vi "Base_Init.vi"(8 "error in (no error)":errorcluster, 10 "String":string, 11 "object in":refnum<class "Base.lvclass">) -> (0 "error out":errorcluster, 3 "object out":refnum<class "Base.lvclass">)   [LabVIEW 2019, in "Base.lvclass"]
uses:
  Base.lvclass
  Base.lvclass/Base.ctl
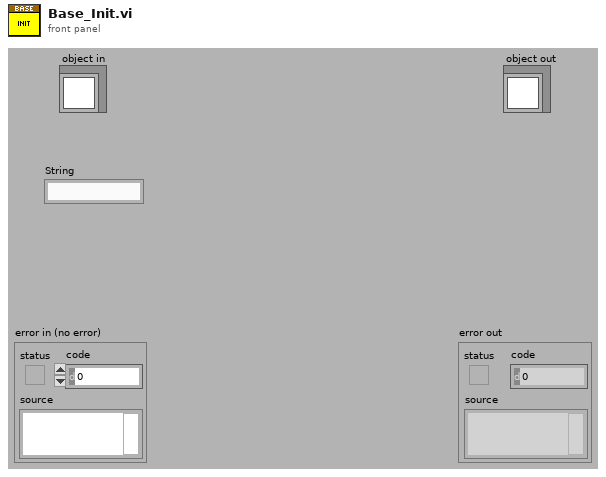
[diagram p1: front panel]
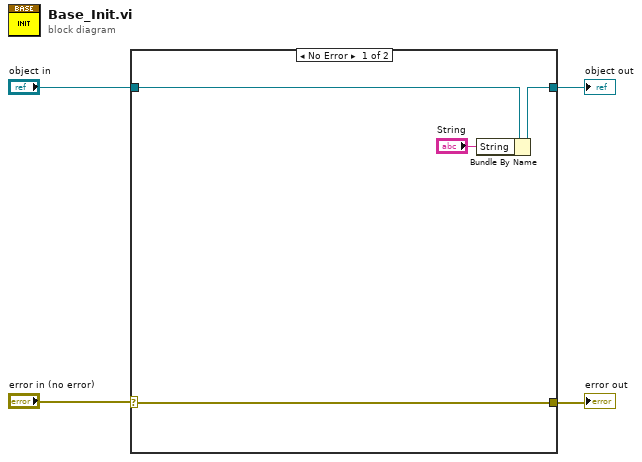
[diagram p0: block diagram]
diagram:
  n1 = case shown="No Error" "error in (no error)" {
    selector: "error in (no error)" -> [w6 w9]
    tunnel: "object in" -> [w8 w10]
    tunnel: [w7 w10] -> w3
    tunnel: [w6 w9] -> w1
    frame No Error {
      n2 = Bundle By Name(cluster=w8, "String"="String") -> (w7:refnum<class "Base.lvclass">)
    }
    frame Error {
    }
  }
  "object out" <- w3
  "error out" <- w1
